vi "sqrtm.vi"(11 "Input Array":dbl[][](array[numeric])) -> (3 "X (sqrt of Matrix)":dbl[][](array[numeric]))   [LabVIEW 2014]
uses:
  <vilib>/Analysis/7linalg.llb/Eigenvalue Order.ctl
  <vilib>/Analysis/7linalg.llb/Real Schur Decomposition.vi
  <vilib>/Analysis/baseanly.llb/Real A x B.vi
  <vilib>/Analysis/baseanly.llb/Complex A x B.vi
  <vilib>/Analysis/Matrix/Comparison/Equal/Equal - RM,RM.vi
  <vilib>/Analysis/Matrix/Numeric/Square Root/Square Root - RM.vi
  <vilib>/Analysis/Matrix/Numeric/Conversions/Matrix To Array - CM.vi
  <vilib>/Analysis/NI_AALPro.lvlib
  <vilib>/Analysis/Matrix/NI_Matrix.lvlib
  <vilib>/Analysis/NI_AALBase.lvlib
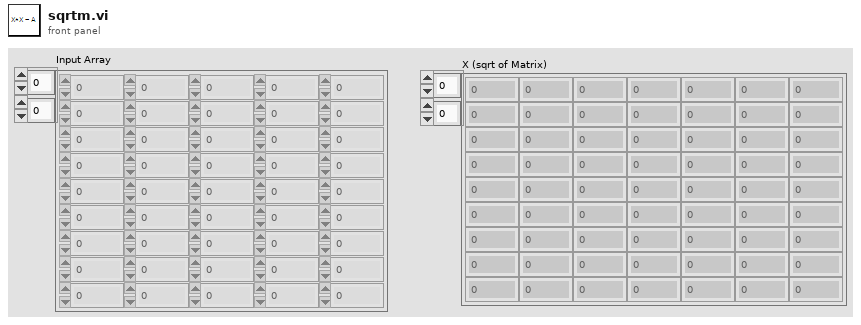
[diagram p1: front panel]
types:
  T1 = typedef "NI_AALPro.lvlib/Eigenvalue Order.ctl" = u16
  T2 = typedef "NI_Matrix.lvlib/RealMatrix.ctl" = dbl[][]
  T3 = typedef "NI_Matrix.lvlib/ComplexMatrix.ctl" = cdb[][]
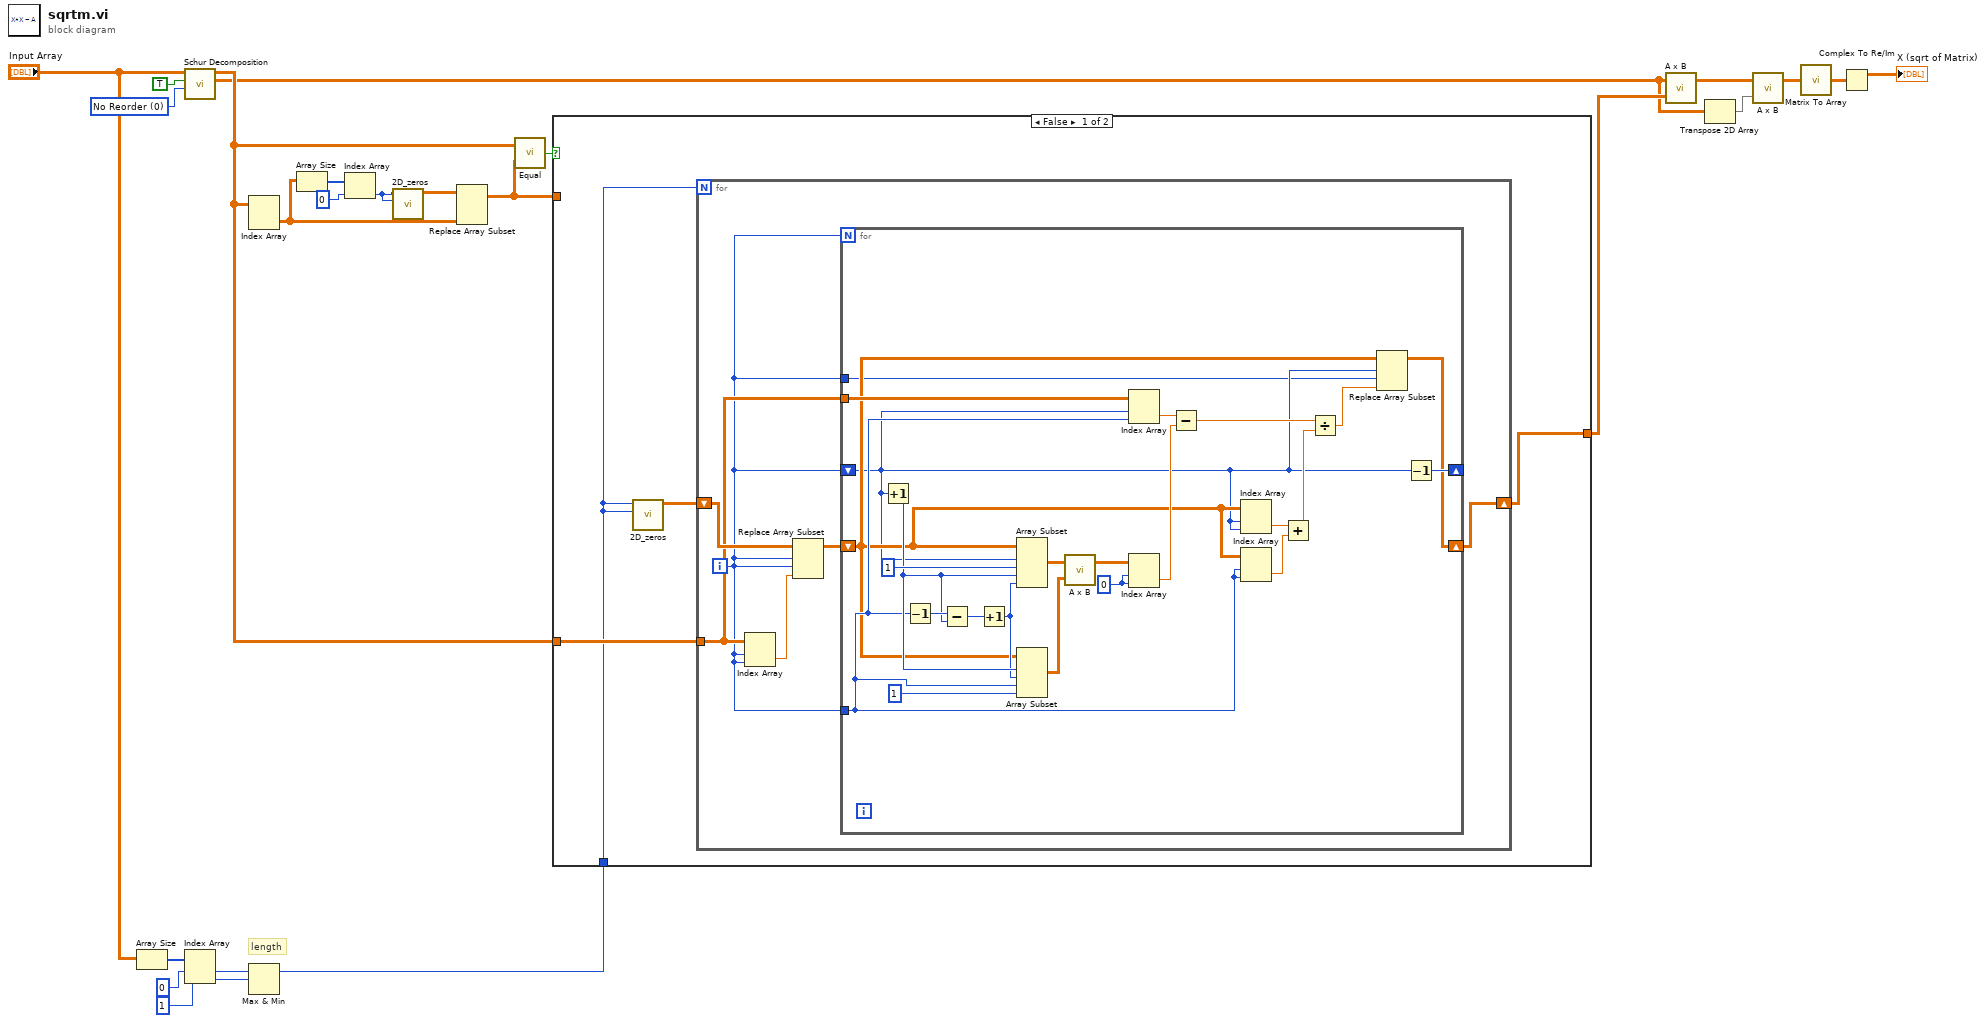
[diagram p0: block diagram]
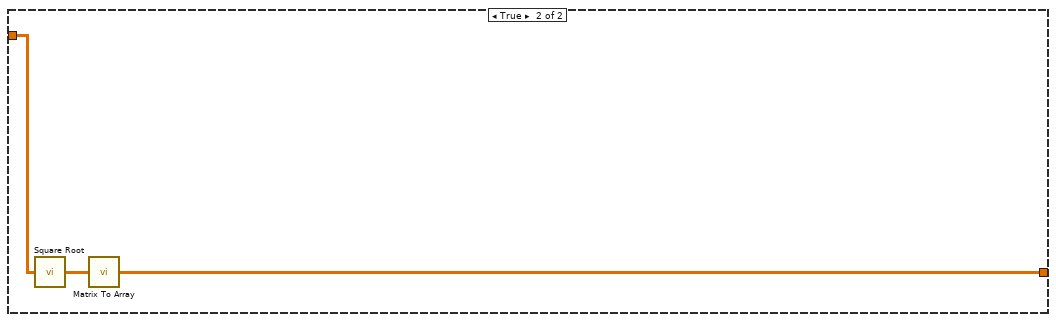
[diagram p2: hidden frame]
diagram:
  w18 = T1 0 items=["No Reorder", "Real Ascending", "Real Descending", "Magnitude Ascending", "Magnitude Descending"] ("order")
  # "length"
  n1 = Array Size(array="Input Array") -> (size(s)=w24:i32[])
  n2 = call-poly <vilib>:"Schur Decomposition.vi"("order"=w18, "compute Schur vectors?"=TRUE, "Input Matrix"="Input Array") -> ("Schur Vectors"=w6:T2, "Schur Form"=w10:T2)  [unwired: 5 in, 2 out]
  n3 = Index Array(array=w24, index #1=0 ("index"), index #2=1 ("index")) -> (element #1=w21:i32, element #2=w20:i32)
  n4 = Index Array(array=w10) -> (element=w17:T2)  [unwired: 2 in]
  n5 = Max & Min(x=w21, y=w20) -> (max(x,y)=w9:i32)  [unwired: 1 out]
  n6 = Array Size(array=w17) -> (size(s)=w15:i32[])
  n7 = Index Array(array=w15, index=0) -> (element=w14:i32)
  n8 = call "2D_zeros.vi"("column_number"=w14, "row_number"=w14) -> ("2D_Rand"=w13:dbl[][])  [unwired: 9 in]
  n9 = Replace Array Subset(array=w13, new element=w17) -> (w11:T2)  [unwired: 2 in]
  n10 = call-poly <vilib>:"Equal.vi"("Real Matrix B"=w11, "Real Matrix A"=w10) -> ("A = B?"=w12:bool)
  n11 = case shown="False" w12 {
    tunnel: w11 -> [_ w61]
    tunnel: [w26 w59] -> w8
    tunnel: w10 -> [w27 _]
    tunnel: w9 -> [w25 _]
    frame False {
      n12 = call "2D_zeros.vi"("column_number"=w25, "row_number"=w25) -> ("2D_Rand"=w28:dbl[][])  [unwired: 9 in]
      n13 = for {
        N: w25 -> [_]
        shift-right: [w29] -> w26
        shift-left: w28 -> [w34]
        tunnel: w27 -> [w31]
        i -> [w30]
        n14 = Index Array(array=w31, index (row)=w30, index (col)=w30) -> (element=w33:dbl)
        n15 = Replace Array Subset(array=w34, new element=w33, index (row)=w30, index (col)=w30) -> (w32:dbl[][])
        n16 = for {
          N: w30 -> [_]
          shift-right: [w58] -> _
          shift-left: w30 -> [w37]
          tunnel: w30 -> [w44]
          tunnel: w31 -> [w47]
          tunnel: w30 -> [w36]
          shift-right: [w35] -> w29
          shift-left: w32 -> [w39]
          w48 = 0 ("length")
          n17 = Increment(x=w37) -> (x+1=w54:i32)
          n18 = Decrement(x=w44) -> (x-1=w55:i32)
          n19 = Subtract(x=w55, y=w54) -> (x-y=w53:i32)
          n20 = Increment(x=w53) -> (x+1=w52:i32)
          n21 = Array Subset(array=w39, index (row)=w37, length (row)=1 ("length"), index (col)=w54, length (col)=w52) -> (w51:dbl[][])
          n22 = Array Subset(array=w39, index (row)=w54, length (row)=w52, index (col)=w44, length (col)=1 ("length")) -> (w50:dbl[][])
          n23 = call-poly <vilib>:"A x B.vi"("B"=w50, "A"=w51) -> ("A x B"=w49:T2)  [unwired: 1 out]
          n24 = Index Array(array=w47, index (row)=w37, index (col)=w44) -> (element=w46:dbl)
          n25 = Index Array(array=w49, index (row)=w48, index (col)=w48) -> (element=w45:dbl)
          n26 = Subtract(x=w46, y=w45) -> (x-y=w41:dbl)
          n27 = Index Array(array=w39, index (row)=w37, index (col)=w37) -> (element=w43:dbl)
          n28 = Index Array(array=w39, index (row)=w44, index (col)=w44) -> (element=w42:dbl)
          n29 = Add(x=w43, y=w42) -> (x+y=w40:dbl)
          n30 = Divide(x=w41, y=w40) -> (x/y=w38:dbl)
          n31 = Replace Array Subset(array=w39, new element=w38, index (row)=w37, index (col)=w36) -> (w35:dbl[][])
          n32 = Decrement(x=w37) -> (x-1=w58:i32)
        }
      }
    }
    frame True {
      n33 = call-poly <vilib>:"Square Root.vi"("Real Matrix A"=w61) -> ("sqrt(A)"=w60:T3)
      n34 = call-poly <vilib>:"Matrix To Array.vi"("Complex Matrix"=w60) -> ("Complex 2D Array"=w59:cdb[][])
    }
  }
  n35 = call-poly <vilib>:"A x B.vi"("B"=w8, "A"=w6) -> ("A x B"=w7:T3)  [unwired: 1 out]
  n36 = Transpose 2D Array(2D array=w6) -> (transposed array=w5:T2)
  n37 = call-poly <vilib>:"A x B.vi"("B"=w5, "A"=w7) -> ("A x B"=w4:T3)  [unwired: 1 out]
  n38 = call-poly <vilib>:"Matrix To Array.vi"("Complex Matrix"=w4) -> ("Complex 2D Array"=w3:cdb[][])
  n39 = Complex To Re/Im(x + iy=w3) -> (x=→"X (sqrt of Matrix)":dbl[][])  [unwired: 1 out]
